vi "PCO_GetMaxLimit.vi"(8 "error in (no error)":errorcluster {"code" format="%x"}, 9 "output_bits":i32, 10 "tint":sgl, 11 "temp":sgl) -> (0 "error out":errorcluster {"code" format="%x"}, 1 "g_max":sgl, 2 "r_max":sgl, 3 "ErrorMessage":i32 format="%x", 5 "b_max":sgl)   [LabVIEW 2020, in "Convert.lvlib"]
doc: "int PCOCONVERT_API PCO_GetMaxLimit(float *r_max, float *g_max, float *b_max, float temp, float tint, int output_bits);"
uses:
  Convert.lvlib
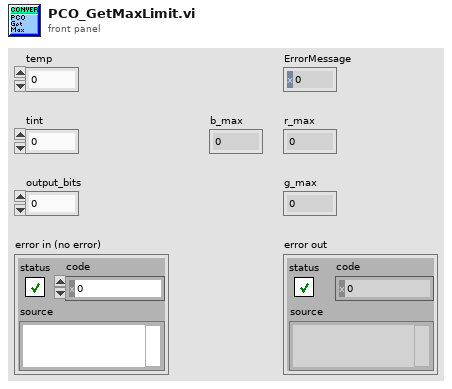
[diagram p1: front panel]
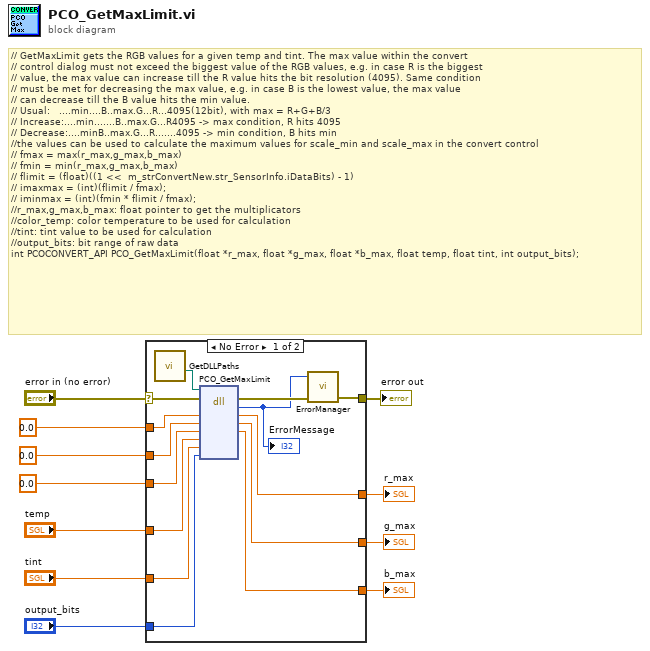
[diagram p0: block diagram]
diagram:
  # "// GetMaxLimit gets the RGB values for a given temp and tint. The max value within the convert\n// control dialog must not exceed the biggest value of the RGB values, e.g. in case R is the biggest\n// value, the max value can increase till the R value hits the bit resolution (4095). Same condition\n// must be met for decreasing the max value, e.g. in case B is the lowest value, the max value\n// can decrease till the B value hits the min value.\n// Usual:   ....min....B..max.G...R...4095(12bit), with max = R+G+B/3\n// Increase:....min.......B..max.G...R4095 -> max condition, R hits 4095\n// Decrease:....minB..max.G...R.......4095 -> min condition, B hits min\n//the values can be used to calculate the maximum values for scale_min and scale_max in the convert control\n// fmax = max(r_max,g_max,b_max)\n// fmin = min(r_max,g_max,b_max)\n// flimit = (float)((1 <<  m_strConvertNew.str_SensorInfo.iDataBits) - 1)\n// imaxmax = (int)(flimit / fmax);\n// iminmax = (int)(fmin * flimit / fmax);\n//r_max,g_max,b_max: float pointer to get the multiplicators\n//color_temp: color temperature to be used for calculation\n//tint: tint value to be used for calculation\n//output_bits: bit range of raw data\nint PCOCONVERT_API PCO_GetMaxLimit(float *r_max, float *g_max, float *b_max, float temp, float tint, int output_bits);"
  n1 = case shown="No Error" "error in (no error)" {
    selector: "error in (no error)" -> [w13 w29]
    tunnel: sgl 0.0 ("r_max") -> [w25 w28]
    tunnel: [w24 w28] -> w10
    tunnel: sgl 0.0 ("g_max") -> [w23 w27]
    tunnel: [w22 w27] -> w8
    tunnel: sgl 0.0 ("b_max") -> [w21 w26]
    tunnel: [w20 w26] -> w6
    tunnel: "temp" -> [w19 _]
    tunnel: "tint" -> [w18 _]
    tunnel: "output_bits" -> [w17 _]
    tunnel: [w15 w29] -> w2
    frame No Error {
      n2 = call "GetDLLPaths.vi"() -> ("PCO_Conv_Path"=w12:path)  [unwired: 9 in, 2 out]
      n3 = dll-call lib="?" fn="PCO_GetMaxLimit"(path in=w12, error in=w13, "r_max"=w25, "g_max"=w23, "b_max"=w21, "temp"=w19, "tint"=w18, "output_bits"=w17) -> (error out=w16:errorcluster, "return type"=w14:i32, "r_max"=w24:sgl, "g_max"=w22:sgl, "b_max"=w20:sgl)  [unwired: 4 in, 1 out]
      "ErrorMessage" <- w14
      n4 = call "ErrorManager.vi"("error in (no error)"=w16, "error code"=w14) -> ("error out"=w15:errorcluster)  [unwired: 3 in]
    }
    frame Error {
    }
  }
  "r_max" <- w10
  "g_max" <- w8
  "b_max" <- w6
  "error out" <- w2
